vi "Poker Hands.vi"(2 "Card Number":dbl) -> (0 "Poker hands Rank and Combination":T1(array[cluster]))   [LabVIEW 2014]
panel:
  out "Rank":i32
  out "Poker hands":string
  out "compare":bool[](array[boolean])
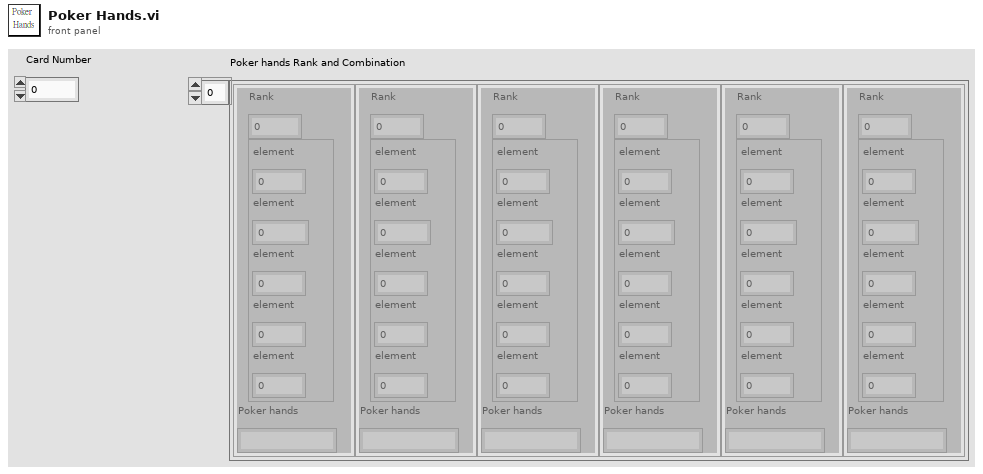
[diagram p1: front panel]
types:
  T1 = cluster{"Rank":i32, cluster{"element":dbl, "element":dbl, "element":dbl, "element":dbl, "element":dbl}, "Poker hands":string}[]
  T2 = cluster{"element":dbl, "element":dbl, "element":dbl, "element":dbl, "element":dbl}[]
  T3 = cluster{"Rank":i32, cluster{"element":dbl, "element":dbl, "element":dbl, "element":dbl, "element":dbl}, "Poker hands":string}
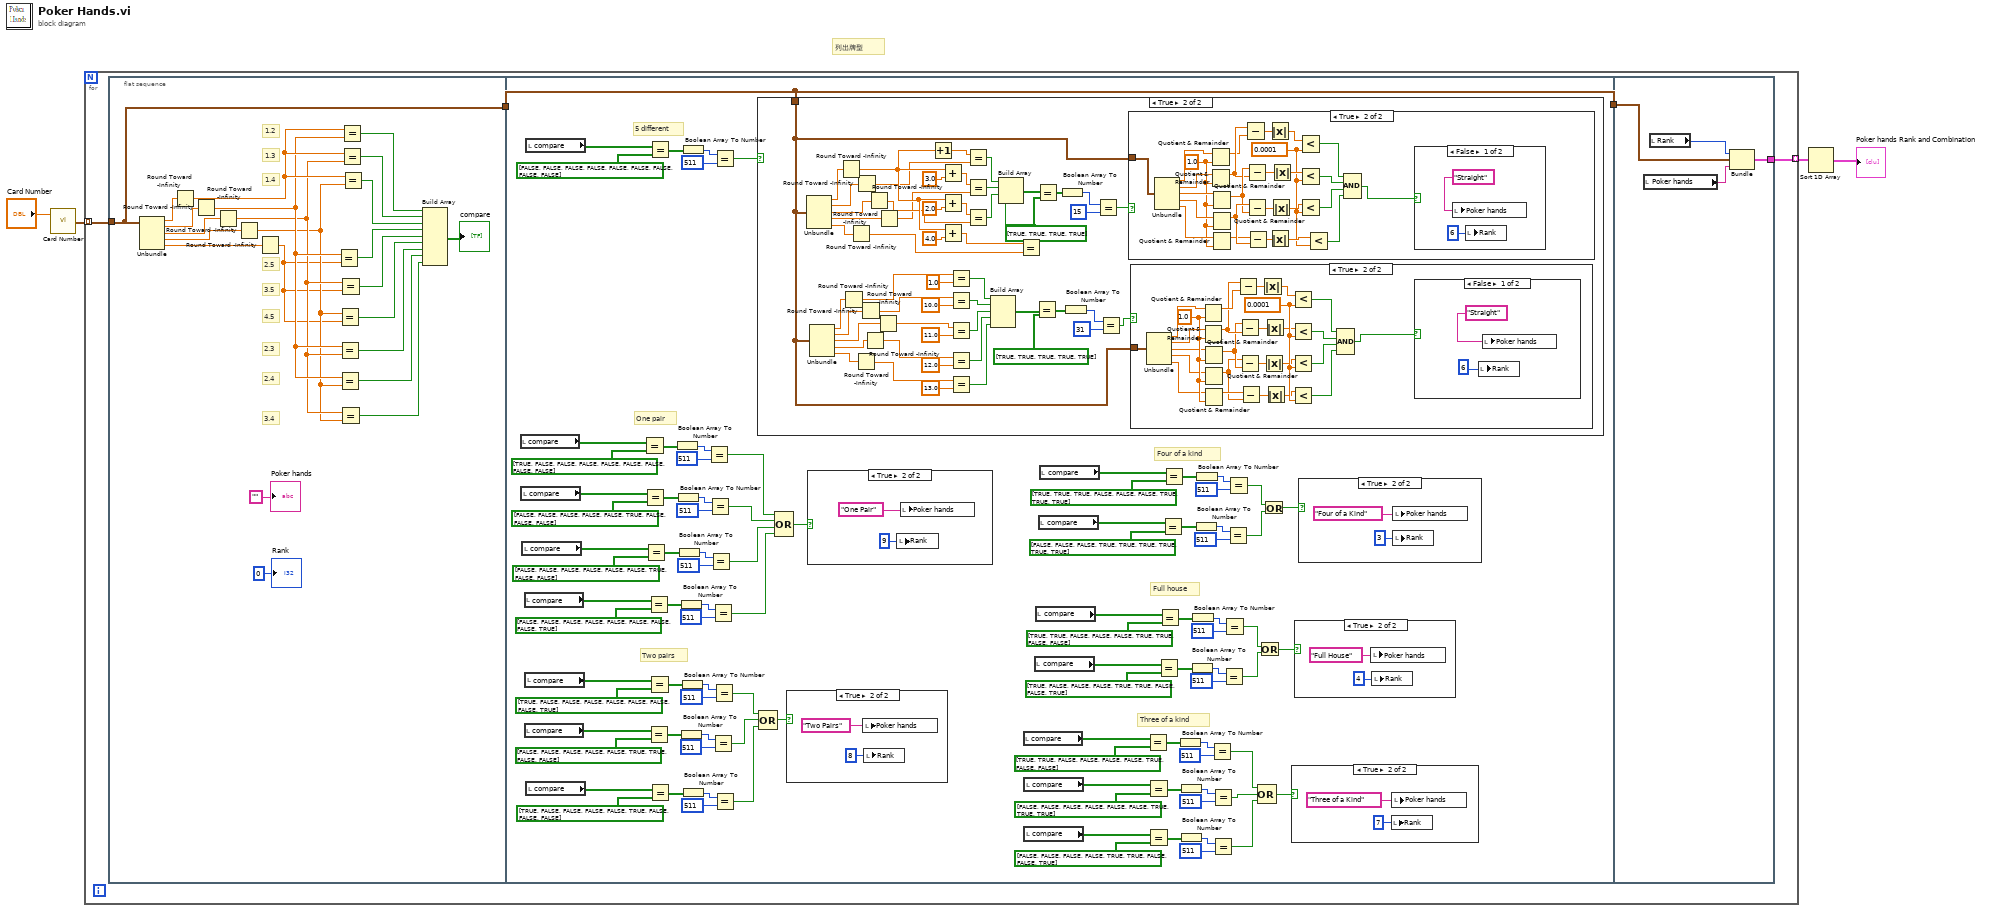
[diagram p0: block diagram]
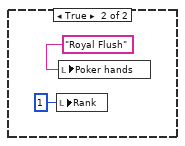
[diagram p9: hidden frame]
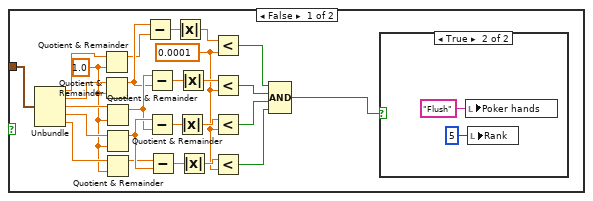
[diagram p10: hidden frame]
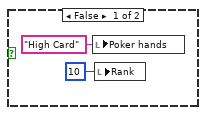
[diagram p11: hidden frame]
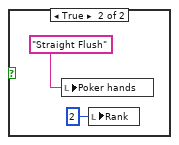
[diagram p12: hidden frame]
diagram:
  # "列出牌型"
  n1 = call "Card Number.vi"("Random Number"="Card Number") -> ("Output"=w3:T2)  [unwired: 1 in]
  n2 = for {
    tunnel: w3 -> [w8] mode=indexing
    tunnel: [w5] -> w2 mode=indexing
    n3 = flat-sequence {
      tunnel: w8 -> [w24]
      tunnel: [w24] -> w7
      tunnel: w7 -> [w45]
      tunnel: [w45] -> w6
      tunnel: w6 -> [w283]
      tunnel: [w282] -> w5
      frame #0 {
        # "3.4"
        # "2.4"
        # "2.3"
        # "4.5"
        # "3.5"
        # "2.5"
        # "1.4"
        # "1.3"
        # "1.2"
        n4 = Unbundle(w24) -> ("element"=w18:dbl, "element"=w16:dbl, "element"=w14:dbl, "element"=w12:dbl, "element"=w10:dbl)
        n5 = Round Toward -Infinity(1:w18) -> (0:w17:dbl)
        n6 = Round Toward -Infinity(1:w16) -> (0:w15:dbl)
        n7 = Round Toward -Infinity(1:w14) -> (0:w13:dbl)
        n8 = Round Toward -Infinity(1:w12) -> (0:w11:dbl)
        n9 = Round Toward -Infinity(1:w10) -> (0:w9:dbl)
        n10 = Equal?(x=w15, y=w9) -> (x = y?=w27:bool)
        n11 = Equal?(x=w11, y=w9) -> (x = y?=w25:bool)
        n12 = Equal?(x=w15, y=w13) -> (x = y?=w21:bool)
        n13 = Equal?(x=w15, y=w11) -> (x = y?=w23:bool)
        n14 = Equal?(x=w13, y=w9) -> (x = y?=w26:bool)
        n15 = Equal?(x=w13, y=w11) -> (x = y?=w22:bool)
        n16 = Equal?(x=w17, y=w15) -> (x = y?=w31:bool)
        n17 = Equal?(x=w17, y=w13) -> (x = y?=w30:bool)
        n18 = Equal?(x=w17, y=w11) -> (x = y?=w29:bool)
        n19 = Build Array(w31, w30, w29, w27, w26, w25, w21, w23, w22) -> (→"compare":bool[])
        "Poker hands" <- ""
        "Rank" <- 0 ("Rank")
      }
      frame #1 {
        # "Four of a kind"
        # "Full house"
        # "Three of a kind"
        # "Two pairs"
        # "One pair"
        # "5 different"
        n20 = local read "compare"() -> (w118:bool[])
        n21 = local read "compare"() -> (w117:bool[])
        n22 = local read "compare"() -> (w108:bool[])
        n23 = local read "compare"() -> (w107:bool[])
        n24 = local read "compare"() -> (w91:bool[])
        n25 = local read "compare"() -> (w92:bool[])
        n26 = local read "compare"() -> (w127:bool[])
        n27 = local read "compare"() -> (w50:bool[])
        n28 = Equal?(x=w118, y=bool[] [TRUE, FALSE, FALSE, FALSE, FALSE, FALSE, FALSE, FALSE, FALSE]) -> (x = y?=w120:bool[])
        n29 = Equal?(x=w117, y=bool[] [FALSE, FALSE, FALSE, FALSE, FALSE, TRUE, FALSE, FALSE, FALSE]) -> (x = y?=w115:bool[])
        n30 = Equal?(x=w108, y=bool[] [FALSE, FALSE, FALSE, FALSE, FALSE, FALSE, TRUE, FALSE, FALSE]) -> (x = y?=w110:bool[])
        n31 = Equal?(x=w107, y=bool[] [FALSE, FALSE, FALSE, FALSE, FALSE, FALSE, FALSE, FALSE, TRUE]) -> (x = y?=w105:bool[])
        n32 = Equal?(x=w91, y=bool[] [FALSE, FALSE, FALSE, FALSE, FALSE, TRUE, TRUE, FALSE, FALSE]) -> (x = y?=w89:bool[])
        n33 = Equal?(x=w92, y=bool[] [TRUE, FALSE, FALSE, FALSE, FALSE, FALSE, FALSE, FALSE, TRUE]) -> (x = y?=w94:bool[])
        n34 = Equal?(x=w127, y=bool[] [FALSE, FALSE, FALSE, FALSE, FALSE, FALSE, FALSE, FALSE, FALSE]) -> (x = y?=w125:bool[])
        n35 = Equal?(x=w50, y=bool[] [TRUE, FALSE, FALSE, FALSE, FALSE, TRUE, FALSE, FALSE, FALSE]) -> (x = y?=w52:bool[])
        n36 = Boolean Array To Number(Boolean array=w120) -> (number=w121:u32)
        n37 = Boolean Array To Number(Boolean array=w115) -> (number=w114:u32)
        n38 = Boolean Array To Number(Boolean array=w110) -> (number=w111:u32)
        n39 = Boolean Array To Number(Boolean array=w105) -> (number=w104:u32)
        n40 = Boolean Array To Number(Boolean array=w89) -> (number=w88:u32)
        n41 = Boolean Array To Number(Boolean array=w94) -> (number=w95:u32)
        n42 = Boolean Array To Number(Boolean array=w125) -> (number=w124:u32)
        n43 = Boolean Array To Number(Boolean array=w52) -> (number=w53:u32)
        n44 = Equal?(x=w121, y=u32 511) -> (x = y?=w102:bool)
        n45 = Equal?(x=w114, y=u32 511) -> (x = y?=w101:bool)
        n46 = Equal?(x=w111, y=u32 511) -> (x = y?=w100:bool)
        n47 = Equal?(x=w104, y=u32 511) -> (x = y?=w99:bool)
        n48 = Equal?(x=w88, y=u32 511) -> (x = y?=w47:bool)
        n49 = Equal?(x=w95, y=u32 511) -> (x = y?=w48:bool)
        n50 = Equal?(x=w124, y=u32 511) -> (x = y?=w98:bool)
        n51 = Equal?(x=w53, y=u32 511) -> (x = y?=w46:bool)
        n52 = case shown="True" w98 {
          tunnel: w45 -> [_ w138]
          frame False {
          }
          frame True {
            n53 = Unbundle(w138) -> ("element"=w159:dbl, "element"=w157:dbl, "element"=w155:dbl, "element"=w151:dbl, "element"=w150:dbl)
            n54 = Unbundle(w138) -> ("element"=w148:dbl, "element"=w146:dbl, "element"=w144:dbl, "element"=w142:dbl, "element"=w140:dbl)
            n55 = Round Toward -Infinity(1:w159) -> (0:w158:dbl)
            n56 = Round Toward -Infinity(1:w148) -> (0:w147:dbl)
            n57 = Round Toward -Infinity(1:w150) -> (0:w149:dbl)
            n58 = Round Toward -Infinity(1:w140) -> (0:w139:dbl)
            n59 = Round Toward -Infinity(1:w157) -> (0:w156:dbl)
            n60 = Round Toward -Infinity(1:w146) -> (0:w145:dbl)
            n61 = Round Toward -Infinity(1:w142) -> (0:w141:dbl)
            n62 = Round Toward -Infinity(1:w155) -> (0:w154:dbl)
            n63 = Round Toward -Infinity(1:w144) -> (0:w143:dbl)
            n64 = Round Toward -Infinity(1:w151) -> (0:w152:dbl)
            n65 = Increment(x=w158) -> (x+1=w191:dbl)
            n66 = Add(x=w158, y=3.0) -> (x+y=w188:dbl)
            n67 = Add(x=w158, y=2.0) -> (x+y=w189:dbl)
            n68 = Add(x=w158, y=4.0) -> (x+y=w185:dbl)
            n69 = Equal?(x=w147, y=1.0) -> (x = y?=w165:bool)
            n70 = Equal?(x=w145, y=10.0) -> (x = y?=w164:bool)
            n71 = Equal?(x=w143, y=11.0) -> (x = y?=w163:bool)
            n72 = Equal?(x=w141, y=12.0) -> (x = y?=w162:bool)
            n73 = Equal?(x=w139, y=13.0) -> (x = y?=w161:bool)
            n74 = Equal?(x=w191, y=w156) -> (x = y?=w184:bool)
            n75 = Equal?(x=w188, y=w152) -> (x = y?=w183:bool)
            n76 = Equal?(x=w189, y=w154) -> (x = y?=w182:bool)
            n77 = Build Array(w165, w164, w163, w162, w161) -> (w166:bool[])
            n78 = Equal?(x=w185, y=w149) -> (x = y?=w181:bool)
            n79 = Build Array(w184, w183, w182, w181) -> (w180:bool[])
            n80 = Equal?(x=w166, y=bool[] [TRUE, TRUE, TRUE, TRUE, TRUE]) -> (x = y?=w168:bool[])
            n81 = Equal?(x=w180, y=bool[] [TRUE, TRUE, TRUE, TRUE]) -> (x = y?=w178:bool[])
            n82 = Boolean Array To Number(Boolean array=w178) -> (number=w177:u32)
            n83 = Boolean Array To Number(Boolean array=w168) -> (number=w169:u32)
            n84 = Equal?(x=w177, y=u32 15) -> (x = y?=w175:bool)
            n85 = Equal?(x=w169, y=u32 31) -> (x = y?=w160:bool)
            n86 = case shown="True" w175 {
              tunnel: w138 -> [w223 w253]
              frame False {
                w230 = 0.0001 ("y")
                w226 = 1.0 ("y")
                n87 = Unbundle(w223) -> ("element"=w224:dbl, "element"=w225:dbl, "element"=w227:dbl, "element"=w228:dbl, "element"=w229:dbl)
                n88 = Quotient & Remainder(x=w224, y=w226) -> (x-y*floor(x/y)=w243:dbl)  [unwired: 1 out]
                n89 = Quotient & Remainder(x=w225, y=w226) -> (x-y*floor(x/y)=w244:dbl)  [unwired: 1 out]
                n90 = Quotient & Remainder(x=w227, y=w226) -> (x-y*floor(x/y)=w245:dbl)  [unwired: 1 out]
                n91 = Quotient & Remainder(x=w228, y=w226) -> (x-y*floor(x/y)=w247:dbl)  [unwired: 1 out]
                n92 = Quotient & Remainder(x=w229, y=w226) -> (x-y*floor(x/y)=w246:dbl)  [unwired: 1 out]
                n93 = Subtract(x=w244, y=w243) -> (x-y=w235:dbl)
                n94 = Subtract(x=w245, y=w244) -> (x-y=w237:dbl)
                n95 = Subtract(x=w247, y=w245) -> (x-y=w239:dbl)
                n96 = Subtract(x=w246, y=w247) -> (x-y=w241:dbl)
                n97 = Absolute Value(x=w235) -> (abs(x)=w236:dbl)
                n98 = Absolute Value(x=w239) -> (abs(x)=w240:dbl)
                n99 = Absolute Value(x=w237) -> (abs(x)=w238:dbl)
                n100 = Absolute Value(x=w241) -> (abs(x)=w242:dbl)
                n101 = Less?(x=w236, y=w230) -> (x < y?=w231:bool)
                n102 = Less?(x=w238, y=w230) -> (x < y?=w232:bool)
                n103 = Less?(x=w240, y=w230) -> (x < y?=w233:bool)
                n104 = Less?(x=w242, y=w230) -> (x < y?=w234:bool)
                n105 = Compound Arithmetic op=AND(w231, w232, w233, w234) -> (w222:bool)
                n106 = case shown="True" w222 {
                  frame False {
                    n107 = local write "Poker hands"("High Card") -> ()
                    n108 = local write "Rank"(10 ("Rank")) -> ()
                  }
                  frame True {
                    n109 = local write "Poker hands"("Flush") -> ()
                    n110 = local write "Rank"(5 ("Rank")) -> ()
                  }
                }
              }
              frame True {
                w260 = 0.0001 ("y")
                w256 = 1.0 ("y")
                n111 = Unbundle(w253) -> ("element"=w254:dbl, "element"=w255:dbl, "element"=w257:dbl, "element"=w258:dbl, "element"=w259:dbl)
                n112 = Quotient & Remainder(x=w254, y=w256) -> (x-y*floor(x/y)=w273:dbl)  [unwired: 1 out]
                n113 = Quotient & Remainder(x=w255, y=w256) -> (x-y*floor(x/y)=w274:dbl)  [unwired: 1 out]
                n114 = Quotient & Remainder(x=w257, y=w256) -> (x-y*floor(x/y)=w275:dbl)  [unwired: 1 out]
                n115 = Quotient & Remainder(x=w258, y=w256) -> (x-y*floor(x/y)=w277:dbl)  [unwired: 1 out]
                n116 = Quotient & Remainder(x=w259, y=w256) -> (x-y*floor(x/y)=w276:dbl)  [unwired: 1 out]
                n117 = Subtract(x=w274, y=w273) -> (x-y=w265:dbl)
                n118 = Subtract(x=w275, y=w274) -> (x-y=w267:dbl)
                n119 = Subtract(x=w277, y=w275) -> (x-y=w269:dbl)
                n120 = Subtract(x=w276, y=w277) -> (x-y=w271:dbl)
                n121 = Absolute Value(x=w265) -> (abs(x)=w266:dbl)
                n122 = Absolute Value(x=w271) -> (abs(x)=w272:dbl)
                n123 = Absolute Value(x=w269) -> (abs(x)=w270:dbl)
                n124 = Absolute Value(x=w267) -> (abs(x)=w268:dbl)
                n125 = Less?(x=w266, y=w260) -> (x < y?=w261:bool)
                n126 = Less?(x=w268, y=w260) -> (x < y?=w262:bool)
                n127 = Less?(x=w270, y=w260) -> (x < y?=w263:bool)
                n128 = Less?(x=w272, y=w260) -> (x < y?=w264:bool)
                n129 = Compound Arithmetic op=AND(w261, w262, w263, w264) -> (w252:bool)
                n130 = case shown="False" w252 {
                  frame False {
                    n131 = local write "Poker hands"("Straight") -> ()
                    n132 = local write "Rank"(6 ("Rank")) -> ()
                  }
                  frame True {
                    n133 = local write "Poker hands"("Straight Flush") -> ()
                    n134 = local write "Rank"(2 ("Rank")) -> ()
                  }
                }
              }
            }
            n135 = case shown="True" w160 {
              tunnel: w138 -> [_ w217]
              frame False {
              }
              frame True {
                w210 = 0.0001 ("y")
                w214 = 1.0 ("y")
                n136 = Unbundle(w217) -> ("element"=w216:dbl, "element"=w215:dbl, "element"=w213:dbl, "element"=w212:dbl, "element"=w211:dbl)
                n137 = Quotient & Remainder(x=w216, y=w214) -> (x-y*floor(x/y)=w197:dbl)  [unwired: 1 out]
                n138 = Quotient & Remainder(x=w215, y=w214) -> (x-y*floor(x/y)=w196:dbl)  [unwired: 1 out]
                n139 = Quotient & Remainder(x=w213, y=w214) -> (x-y*floor(x/y)=w195:dbl)  [unwired: 1 out]
                n140 = Quotient & Remainder(x=w212, y=w214) -> (x-y*floor(x/y)=w193:dbl)  [unwired: 1 out]
                n141 = Quotient & Remainder(x=w211, y=w214) -> (x-y*floor(x/y)=w194:dbl)  [unwired: 1 out]
                n142 = Subtract(x=w196, y=w197) -> (x-y=w205:dbl)
                n143 = Subtract(x=w195, y=w196) -> (x-y=w203:dbl)
                n144 = Subtract(x=w193, y=w195) -> (x-y=w201:dbl)
                n145 = Subtract(x=w194, y=w193) -> (x-y=w199:dbl)
                n146 = Absolute Value(x=w205) -> (abs(x)=w204:dbl)
                n147 = Absolute Value(x=w201) -> (abs(x)=w200:dbl)
                n148 = Absolute Value(x=w203) -> (abs(x)=w202:dbl)
                n149 = Absolute Value(x=w199) -> (abs(x)=w198:dbl)
                n150 = Less?(x=w204, y=w210) -> (x < y?=w209:bool)
                n151 = Less?(x=w202, y=w210) -> (x < y?=w208:bool)
                n152 = Less?(x=w200, y=w210) -> (x < y?=w207:bool)
                n153 = Less?(x=w198, y=w210) -> (x < y?=w206:bool)
                n154 = Compound Arithmetic op=AND(w209, w208, w207, w206) -> (w192:bool)
                n155 = case shown="False" w192 {
                  frame False {
                    n156 = local write "Rank"(6 ("Rank")) -> ()
                    n157 = local write "Poker hands"("Straight") -> ()
                  }
                  frame True {
                    n158 = local write "Rank"(1 ("Rank")) -> ()
                    n159 = local write "Poker hands"("Royal Flush") -> ()
                  }
                }
              }
            }
          }
        }
        n160 = Compound Arithmetic op=OR(w48, w47, w46) -> (w49:bool)
        n161 = Compound Arithmetic op=OR(w102, w101, w100, w99) -> (w97:bool)
        n162 = case shown="True" w49 {
          frame False {
          }
          frame True {
            n163 = local write "Poker hands"("Two Pairs") -> ()
            n164 = local write "Rank"(8 ("Rank")) -> ()
          }
        }
        n165 = case shown="True" w97 {
          frame False {
          }
          frame True {
            n166 = local write "Rank"(9 ("Rank")) -> ()
            n167 = local write "Poker hands"("One Pair") -> ()
          }
        }
        n168 = local read "compare"() -> (w82:bool[])
        n169 = local read "compare"() -> (w81:bool[])
        n170 = local read "compare"() -> (w72:bool[])
        n171 = local read "compare"() -> (w60:bool[])
        n172 = local read "compare"() -> (w59:bool[])
        n173 = local read "compare"() -> (w39:bool[])
        n174 = local read "compare"() -> (w40:bool[])
        n175 = Equal?(x=w82, y=bool[] [TRUE, TRUE, FALSE, FALSE, FALSE, FALSE, TRUE, FALSE, FALSE]) -> (x = y?=w84:bool[])
        n176 = Equal?(x=w81, y=bool[] [FALSE, FALSE, FALSE, FALSE, FALSE, FALSE, TRUE, TRUE, TRUE]) -> (x = y?=w79:bool[])
        n177 = Equal?(x=w72, y=bool[] [FALSE, FALSE, FALSE, FALSE, TRUE, TRUE, FALSE, FALSE, TRUE]) -> (x = y?=w74:bool[])
        n178 = Equal?(x=w60, y=bool[] [TRUE, FALSE, FALSE, FALSE, TRUE, TRUE, FALSE, FALSE, TRUE]) -> (x = y?=w62:bool[])
        n179 = Equal?(x=w59, y=bool[] [TRUE, TRUE, FALSE, FALSE, FALSE, TRUE, TRUE, FALSE, FALSE]) -> (x = y?=w57:bool[])
        n180 = Equal?(x=w39, y=bool[] [FALSE, FALSE, FALSE, TRUE, TRUE, TRUE, TRUE, TRUE, TRUE]) -> (x = y?=w37:bool[])
        n181 = Equal?(x=w40, y=bool[] [TRUE, TRUE, TRUE, FALSE, FALSE, FALSE, TRUE, TRUE, TRUE]) -> (x = y?=w42:bool[])
        n182 = Boolean Array To Number(Boolean array=w84) -> (number=w85:u32)
        n183 = Boolean Array To Number(Boolean array=w79) -> (number=w78:u32)
        n184 = Boolean Array To Number(Boolean array=w74) -> (number=w75:u32)
        n185 = Boolean Array To Number(Boolean array=w62) -> (number=w63:u32)
        n186 = Boolean Array To Number(Boolean array=w57) -> (number=w56:u32)
        n187 = Boolean Array To Number(Boolean array=w37) -> (number=w36:u32)
        n188 = Boolean Array To Number(Boolean array=w42) -> (number=w43:u32)
        n189 = Equal?(x=w85, y=u32 511) -> (x = y?=w71:bool)
        n190 = Equal?(x=w78, y=u32 511) -> (x = y?=w70:bool)
        n191 = Equal?(x=w75, y=u32 511) -> (x = y?=w69:bool)
        n192 = Equal?(x=w63, y=u32 511) -> (x = y?=w66:bool)
        n193 = Equal?(x=w56, y=u32 511) -> (x = y?=w65:bool)
        n194 = Equal?(x=w36, y=u32 511) -> (x = y?=w33:bool)
        n195 = Equal?(x=w43, y=u32 511) -> (x = y?=w34:bool)
        n196 = Or(x=w65, y=w66) -> (x .or. y?=w67:bool)
        n197 = Compound Arithmetic op=OR(w71, w70, w69) -> (w68:bool)
        n198 = Or(x=w34, y=w33) -> (x .or. y?=w32:bool)
        n199 = case shown="True" w68 {
          frame False {
          }
          frame True {
            n200 = local write "Rank"(7 ("Rank")) -> ()
            n201 = local write "Poker hands"("Three of a Kind") -> ()
          }
        }
        n202 = case shown="True" w67 {
          frame False {
          }
          frame True {
            n203 = local write "Poker hands"("Full House") -> ()
            n204 = local write "Rank"(4 ("Rank")) -> ()
          }
        }
        n205 = case shown="True" w32 {
          frame False {
          }
          frame True {
            n206 = local write "Poker hands"("Four of a Kind") -> ()
            n207 = local write "Rank"(3 ("Rank")) -> ()
          }
        }
      }
      frame #2 {
        n208 = local read "Poker hands"() -> (w285:string)
        n209 = local read "Rank"() -> (w284:i32)
        n210 = Bundle("Rank"=w284, w283, "Poker hands"=w285) -> (w282:T3)  [unwired: 1 in]
      }
    }
  }
  n211 = Sort 1D Array(array=w2) -> (sorted array=→"Poker hands Rank and Combination":T1)
